vi "Get Size.vi"(8 "error in (no error)":errorcluster, 11 "Array1D in":refnum<class "Array1D.lvclass">) -> (0 "error out":errorcluster, 2 "Size":i32, 3 "Array1D out":refnum<class "Array1D.lvclass">)   [LabVIEW 2021, in "Array1D.lvclass"]
uses:
  Array1D.lvclass
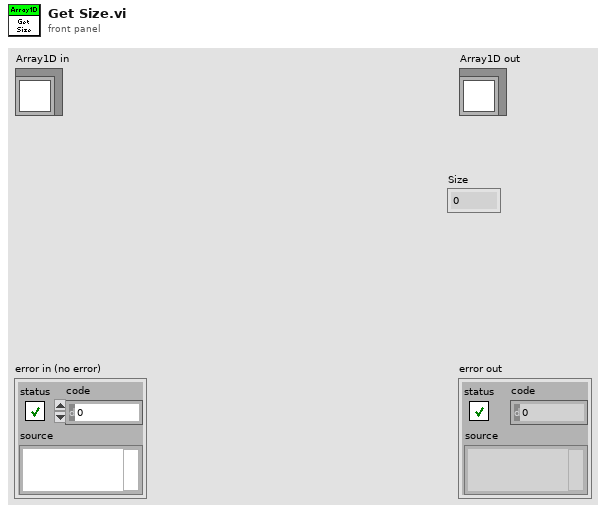
[diagram p1: front panel]
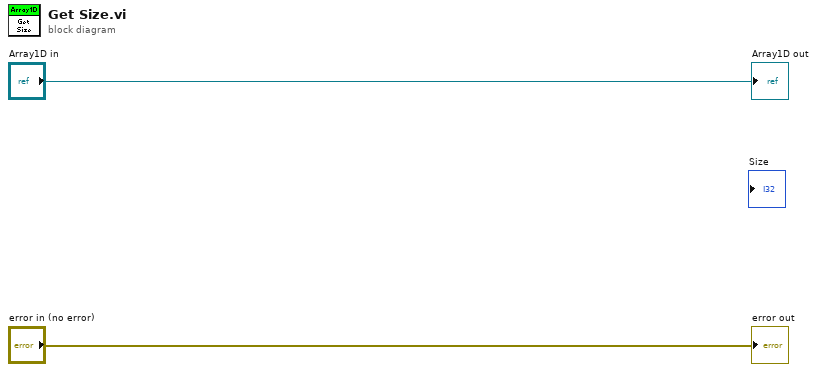
[diagram p0: block diagram]
diagram:
  "error out" <- "error in (no error)"
  "Array1D out" <- "Array1D in"
